vi "Demo_Index.vi"(11 "Index IN":i32) -> (2 "Trig0/Ack1":i32, 3 "Station number":i32)   [LabVIEW 2017]
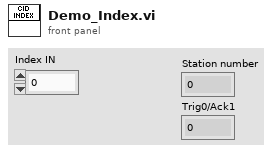
[diagram p1: front panel]
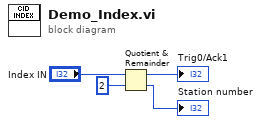
[diagram p0: block diagram]
diagram:
  n1 = Quotient & Remainder(x="Index IN", y=2) -> (x-y*floor(x/y)=→"Trig0/Ack1":i32, floor(x/y)=→"Station number":i32)
